vi "Noise Waveforms and PS Density.vi"() -> ()   [LabVIEW 2023]
doc: "Generates a signal with a large amount of noise, then calculates the power spectrum."
uses:
  <vilib>/Analysis/4window.llb/windowTd.ctl
  <vilib>/measure/maspectr.llb/Power Spectrum and PSD Export Mode.ctl
  <vilib>/measure/maspectr.llb/FFT Power Spectrum and PSD for 1 Chan.vi
  <vilib>/measure/NI_MABase.lvlib
  <vilib>/measure/NI_MAPro.lvlib
  <vilib>/Analysis/NI_AALPro.lvlib
panel:
  in  "Stop":bool
  in  "noise amplitude":dbl=0.1 format="%#.6g"
  in  "noise type":T1(ring)=enum."inverse f"
  out "Power Spectral Density":cluster{"f0":dbl, "df":dbl, "magnitude":dbl[]}(graph)
  in  "sine amplitude":dbl=1.0 format="%#.6g"
  in  "sine frequency":dbl=1.0 format="%#.6g"
  in  "sampling info":cluster{"Fs":dbl, "#s":dbl}={"Fs"=1000.0, "#s"=10000.0} {"#s" format="%#.6g"; "Fs" format="%#.6g"}
  out "Waveform":waveform(dbl)(graph)
  # "Overview: Demonstrates the power spectral density profiles of a variety of noise sources.\nRequirements: LabVIEW Full Development System\nInstructions:\n1. Run the VI.\n2. Select the noise type and note the shape of the selected noise in the Power Spectral Density graph.\n3. Click Stop to stop the VI."
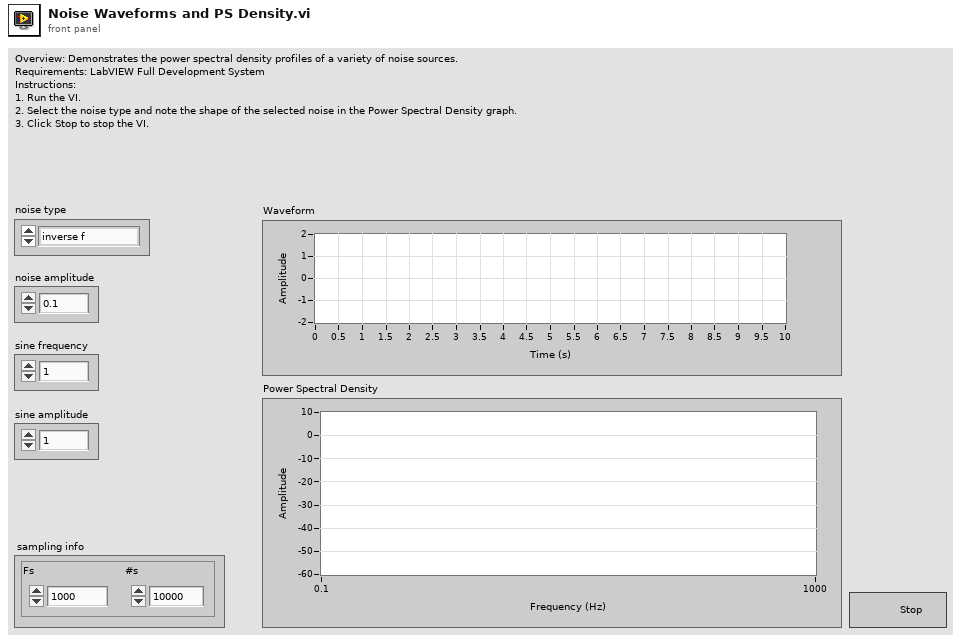
[diagram p1: front panel]
types:
  T1 = enum16{"uniform white", "Gaussian white", "periodic", "inverse f"}
  T2 = cluster{"averaging mode":enum16{"No averaging", "Vector averaging", "RMS averaging", "Peak hold"}, "weighting mode":enum16{"Linear", "Exponential"}, "number of averages":u32}
  T3 = cluster{"lower cutoff freq":dbl, "higher cutoff freq":dbl, "order":i32}
  T4 = typedef "NI_MAPro.lvlib/Power Spectrum and PSD Export Mode.ctl" = u16
  T5 = typedef "NI_AALPro.lvlib/windowTd.ctl" = u32
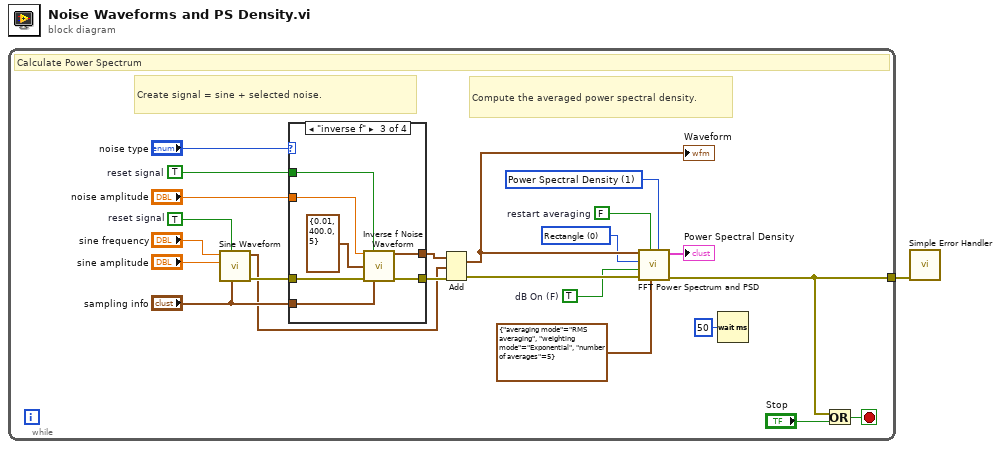
[diagram p0: block diagram]
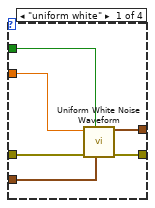
[diagram p2: hidden frame]
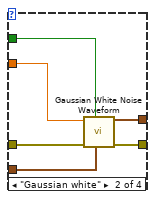
[diagram p3: hidden frame]
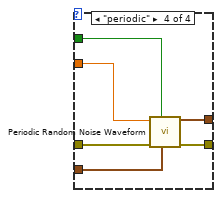
[diagram p4: hidden frame]
diagram:
  n1 = while {
    tunnel: [w3] -> w1
    stop <- w4 stop-if-true
    w5 = T4 1 items=["Power Spectrum", "Power Spectral Density"] ("export mode")
    w6 = T5 0 items=["Rectangle"=0, "Hanning"=1, "Hamming"=2, "Blackman-Harris"=3, "Exact Blackman"=4, "Blackman"=5, "Flat Top"=6, "4 Term B-Harris "=7, "7 Term B-Harris"=8, "Low Sidelobe"=9, "Blackman Nuttall"=11, "Triangle"=30, "Bartlett-Hanning"=31, "Bohman"=32, "Parzen"=33, "Welch"=34, "Kaiser"=60, "Dolph-Chebyshev"=61, "Gaussian"=62] ("window")
    w18 = TRUE  # reset signal
    w21 = FALSE  # restart averaging
    w7 = TRUE  # dB On (F)
    w24 = TRUE  # reset signal
    # "Compute the averaged power spectral density."
    # "Create signal = sine + selected noise."
    # "Calculate Power Spectrum"
    n2 = call <vilib>:"Sine Waveform.vi"("sampling info"="sampling info", "reset signal"=w24, "amplitude"="sine amplitude", "frequency"="sine frequency") -> ("error out"=w20:errorcluster, "signal out"=w13:waveform(dbl))  [unwired: 6 in]
    n3 = case shown="\"inverse f\"" "noise type" {
      tunnel: w20 -> [w30 w36 w43 w49]
      tunnel: "sampling info" -> [w29 w35 w42 w48]
      tunnel: w18 -> [w28 w34 w41 w44]
      tunnel: "noise amplitude" -> [w27 w33 w40 w47]
      tunnel: [w26 w32 w39 w46] -> w14
      tunnel: [w25 w31 w38 w45] -> w15
      frame "uniform white" {
        n4 = call <vilib>:"Uniform White Noise Waveform.vi"("sampling info"=w29, "reset signal"=w28, "error in (no error)"=w30, "amplitude"=w27) -> ("error out"=w25:errorcluster, "signal out"=w26:waveform(dbl))  [unwired: 6 in]
      }
      frame "Gaussian white" {
        n5 = call <vilib>:"Gaussian White Noise Waveform.vi"("sampling info"=w35, "reset signal"=w34, "error in (no error)"=w36, "standard deviation"=w33) -> ("error out"=w31:errorcluster, "signal out"=w32:waveform(dbl))  [unwired: 6 in]
      }
      frame "inverse f" {
        n6 = call <vilib>:"Inverse f Noise Waveform.vi"("noise density"=w40, "reset signal (F)"=w41, "filter specifications"=T3 {"lower cutoff freq"=0.01, "higher cutoff freq"=400.0, "order"=5}, "error in (no error)"=w43, "sampling info"=w42) -> ("signal out"=w39:waveform(dbl), "error out"=w38:errorcluster)  [unwired: 6 in, 3 out]
      }
      frame "periodic" {
        n7 = call <vilib>:"Periodic Random Noise Waveform.vi"("sampling info"=w48, "reset signal"=w44, "error in (no error)"=w49, "spectral amplitude"=w47) -> ("error out"=w45:errorcluster, "signal out"=w46:waveform(dbl))  [unwired: 6 in]
      }
    }
    n8 = Add(1:w13, 2:w14, 4:w15) -> (0:w11:waveform(dbl), 3:w12:errorcluster)
    "Waveform" <- w11
    n9 = call-poly <vilib>:"FFT Power Spectrum and PSD.vi"("export mode"=w5, "averaging parameters"=T2 {"averaging mode"=enum."RMS averaging", "weighting mode"=enum."Exponential", "number of averages"=5}, "restart averaging (F)"=w21, "error in (no error)"=w12, "dB On (F)"=w7, "window"=w6, "time signal"=w11) -> ("error out"=w3:errorcluster, "Power Spectrum / PSD"=→"Power Spectral Density":cluster{"f0":dbl, "df":dbl, "magnitude":dbl[]})  [unwired: 1 in, 2 out]
    n10 = Wait (ms)(milliseconds to wait=u32 50) -> ()  [unwired: 1 out]
    n11 = Or(x=w3, y="Stop") -> (x .or. y?=w4:bool)
  }
  n12 = call <vilib>:"Simple Error Handler.vi"("error in (no error)"=w1) -> ()  [unwired: 4 in, 5 out]
